vi "SC TCP Unflatten SoundCheck Status.vi"(8 "error in":errorcluster, 11 "Response JSON":string) -> (0 "error out":errorcluster, 3 "Return":T1)   [LabVIEW 2018]
uses:
  SC TCP SoundCheckStatus.ctl
panel:
  out "Command Completed":bool
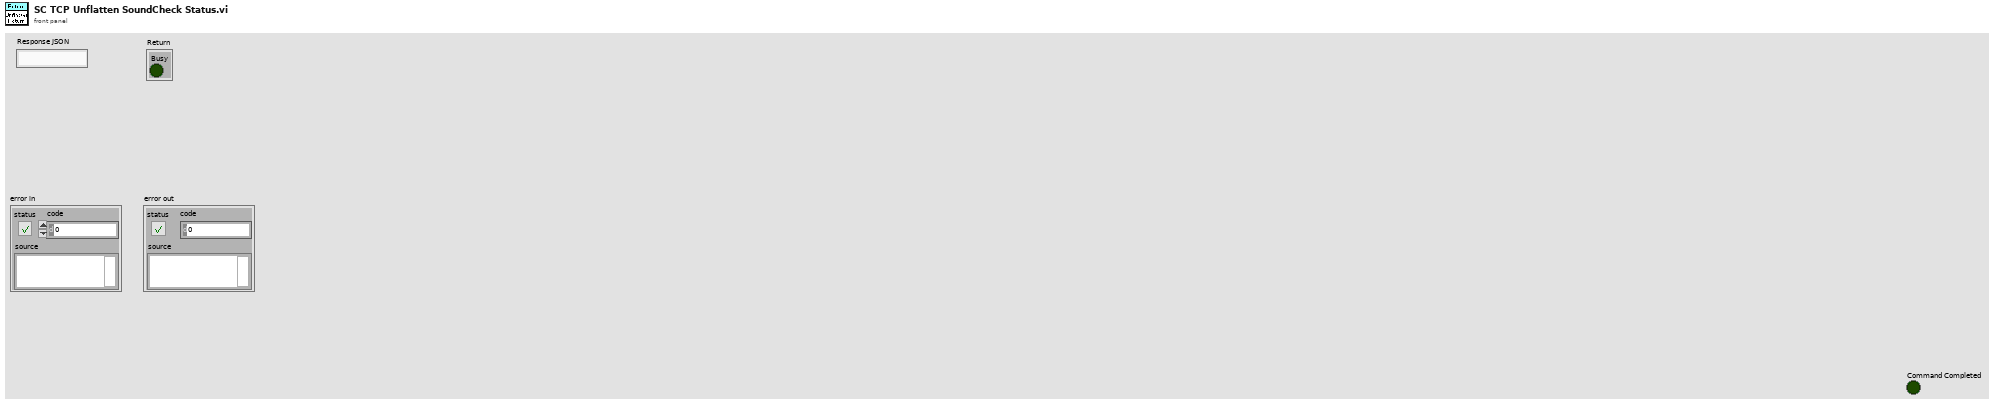
[diagram p1: front panel]
types:
  T1 = typedef "SC TCP SoundCheckStatus.ctl" = cluster{"Busy":bool}
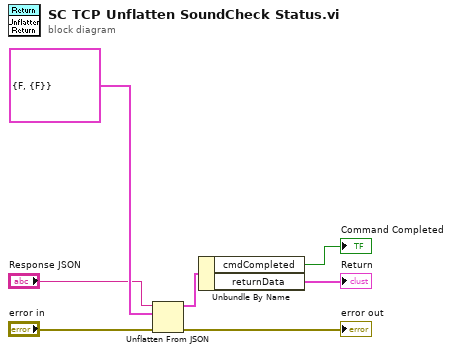
[diagram p0: block diagram]
diagram:
  n1 = Unflatten From JSON(JSON string="Response JSON", type and defaults=cluster{"cmdCompleted":bool, "returnData":T1} {"cmdCompleted"=FALSE, "returnData"={"Busy"=FALSE}} ("Response Details"), error in (no error)="error in") -> (value=w6:cluster{"cmdCompleted":bool, "returnData":T1}, error out=→"error out":errorcluster)  [unwired: 4 in]
  n2 = Unbundle By Name(w6) -> ("cmdCompleted"=→"Command Completed":bool, "returnData"=→"Return":T1)
